vi "WriteDataToTextFile.vi"(4 "number of points/acquisition":i32=10, 5 "number of acquisitions":i32=10, 6 "Byte Stream File Refnum":refnum<file>) -> (0 "error out":errorcluster, 2 "Array Data":string[](array[string]))   [LabVIEW 2012]
panel:
  in  "error in (no error)":errorcluster
  out "data":sgl[](graph)
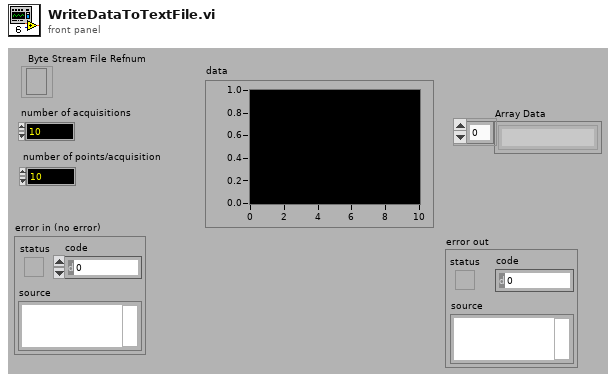
[diagram p1: front panel]
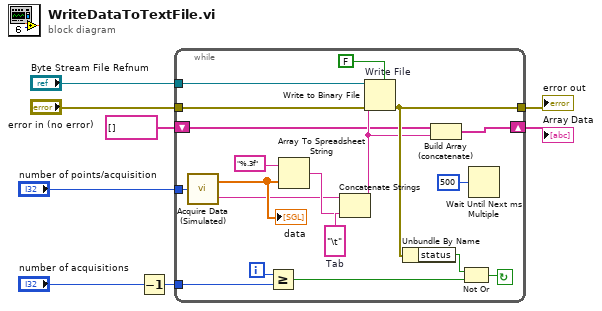
[diagram p0: block diagram]
diagram:
  n1 = Decrement(x="number of acquisitions") -> (x-1=w6:i32)
  n2 = while {
    tunnel: "Byte Stream File Refnum" -> [w15]
    tunnel: [w14] -> w4
    tunnel: w6 -> [w21]
    tunnel: "error in (no error)" -> [w16]
    tunnel: "number of points/acquisition" -> [w27]
    shift-right: [w11] -> w1
    shift-left: string[] [] -> [w10]
    i -> [w22]
    stop <- w20 continue-if-true
    w26 = "\t"  # Tab
    n3 = call "Acquire Data (Simulated).vi"("# of points"=w27) -> ("data"=w18:sgl[], "time"=w17:string)
    "data" <- w18
    n4 = Greater Or Equal?(x=w22, y=w21) -> (x >= y?=w23:bool)
    n5 = Array To Spreadsheet String(array=w18, 3:"%.3f") -> (spreadsheet string=w25:string)  [unwired: 1 out]
    n6 = Concatenate Strings(w17, w26, w25) -> (w12:string)
    n7 = Write to Binary File "Write File"(file (use dialog)=w15, data=w12, error in=w16, 5:FALSE ("prepend array or string size? (T)")) -> (error out=w14:errorcluster)  [unwired: 4 out]
    n8 = Unbundle By Name(w14) -> ("status"=w24:bool)
    n9 = Build Array (concatenate)(w10, w12) -> (w11:string[])
    n10 = Not Or(1:w23, 2:w24) -> (0:w20:bool)
    n11 = Wait Until Next ms Multiple(millisecond multiple=u32 500) -> ()  [unwired: 1 out]
  }
  "error out" <- w4
  "Array Data" <- w1
